vi "Reinitialize All.vi"(8 "error in (no error)":errorcluster, 10 "Initialize Hot And Cold Source Unit":bool, 11 "Hot And Cold Source Unit View in":refnum<class "Hot And Cold Source Unit View.lvclass">) -> (0 "error out":errorcluster, 3 "Hot And Cold Source Unit View out":refnum<class "Hot And Cold Source Unit View.lvclass">)   [LabVIEW 2013, in "Hot And Cold Source Unit View.lvlib" / "Hot And Cold Source Unit View.lvclass"]
uses:
  Hot And Cold Source Unit View.lvclass
  Hot And Cold Source Unit View.lvclass/Hot And Cold Source Unit View.ctl
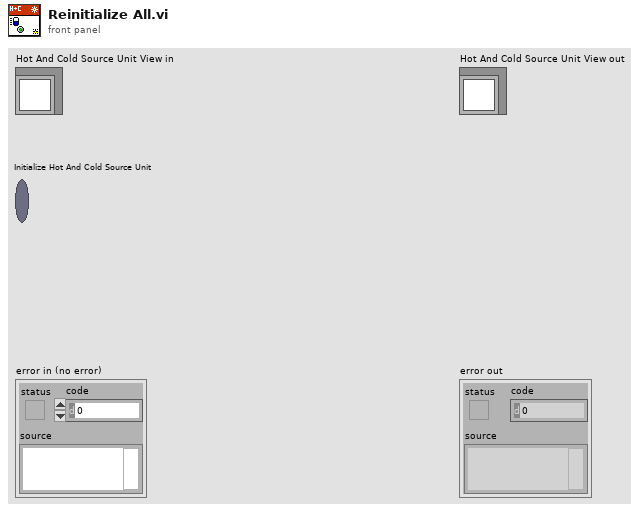
[diagram p1: front panel]
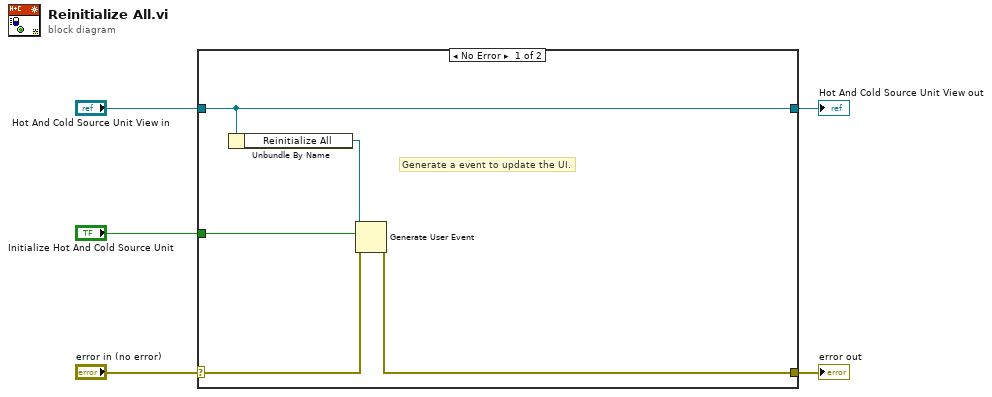
[diagram p0: block diagram]
diagram:
  n1 = case shown="No Error" "error in (no error)" {
    selector: "error in (no error)" -> [w7 w12]
    tunnel: [w6 w12] -> w4
    tunnel: [w10 w11] -> w2
    tunnel: "Hot And Cold Source Unit View in" -> [w10 w11]
    tunnel: "Initialize Hot And Cold Source Unit" -> [w8 _]
    frame No Error {
      # "Generate a event to update the UI."
      n2 = Unbundle By Name(w10) -> ("Reinitialize All"=w9:refnum<user-event>)
      n3 = Generate User Event(user event=w9, event data cluster=w8, error in=w7) -> (error out=w6:errorcluster)  [unwired: 1 in, 1 out]
    }
    frame Error {
    }
  }
  "error out" <- w4
  "Hot And Cold Source Unit View out" <- w2
